vi "Dispense.vi"(0 "reference in":refnum<class "Gum Machine.lvclass">, 5 "error in (no error)":errorcluster) -> (14 "reference out":refnum<class "Gum Machine.lvclass">, 19 "error out":errorcluster)   [LabVIEW 2013]
uses:
  Gum Machine.lvclass
  State_class/State.lvclass
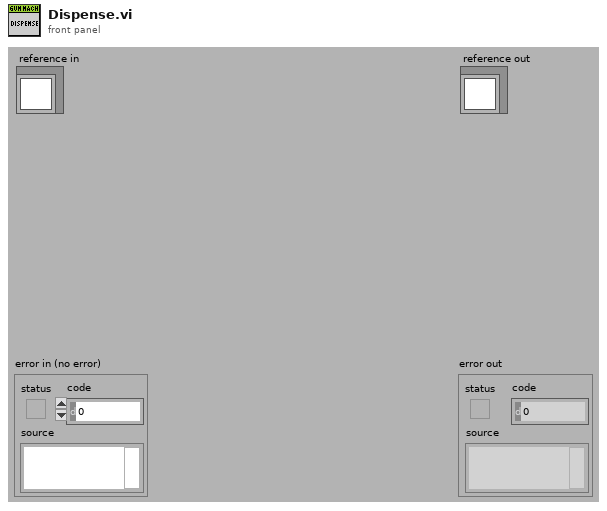
[diagram p1: front panel]
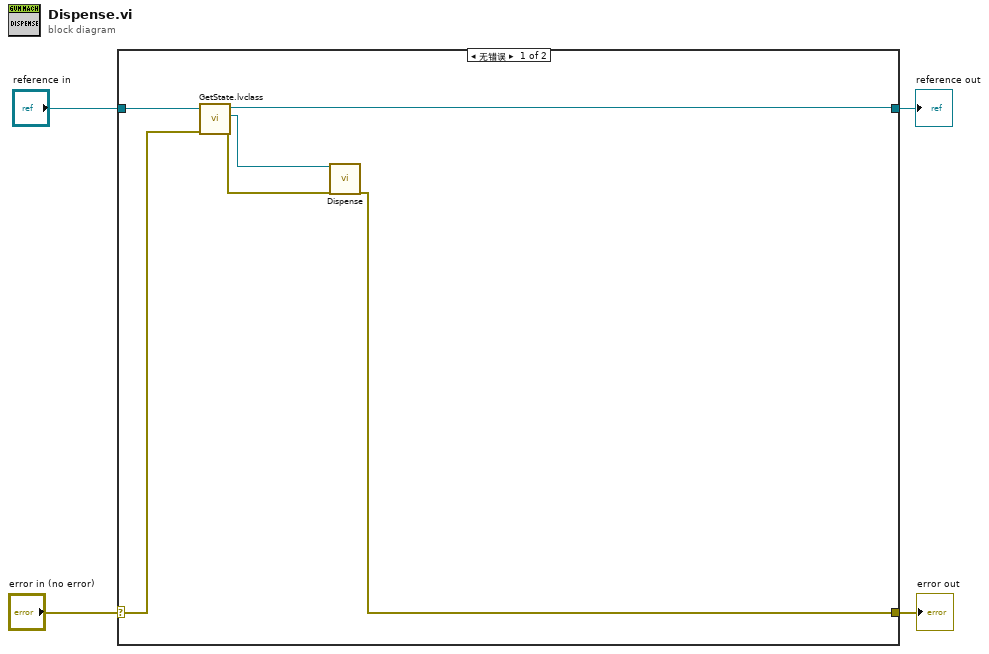
[diagram p0: block diagram]
diagram:
  n1 = case shown="无错误" "error in (no error)" {
    selector: "error in (no error)" -> [w7 w12]
    tunnel: [w5 w12] -> w3
    tunnel: [w9 w11] -> w1
    tunnel: "reference in" -> [w10 w11]
    frame No Error {
      n2 = call-dynamic "GetState.lvclass.vi"("error in (no error)"=w7, "reference in"=w10) -> ("error out"=w6:errorcluster, "State.lvclass"=w8:refnum<class "State.lvclass">, "reference out"=w9:refnum<class "Gum Machine.lvclass">)  [unwired: 7 in]
      n3 = call-dynamic "Dispense.vi"("reference in"=w8, "error in (no error)"=w6) -> ("error out"=w5:errorcluster)  [unwired: 16 in, 1 out]
    }
    frame Error {
    }
  }
  "error out" <- w3
  "reference out" <- w1
